vi "daq.vi"() -> ()   [LabVIEW 2010]
panel:
  in  "Array?":bool
  in  "Input":dbl format="%0.2f"
  in  "Tab Control":enum32{"DAQ"}(tab)
  out "Waveform DAQ":waveform(dbl)(graph)
  in  "Calibracion DAQ":T1
  in  "DAQ Controls":T2={"Minimum Value"=-10.0, "Maximum Value"=10.0, "Physical Channel"="Dev1/ao0", "DAQ Fs (S/s)"=10000.0} {"Minimum Value" min=-10.0 max=0.0; "Maximum Value" min=0.0 max=10.0}
  in  "tiempo (ms)":dbl
  in  "DAQ?":bool
  in  "stop":bool
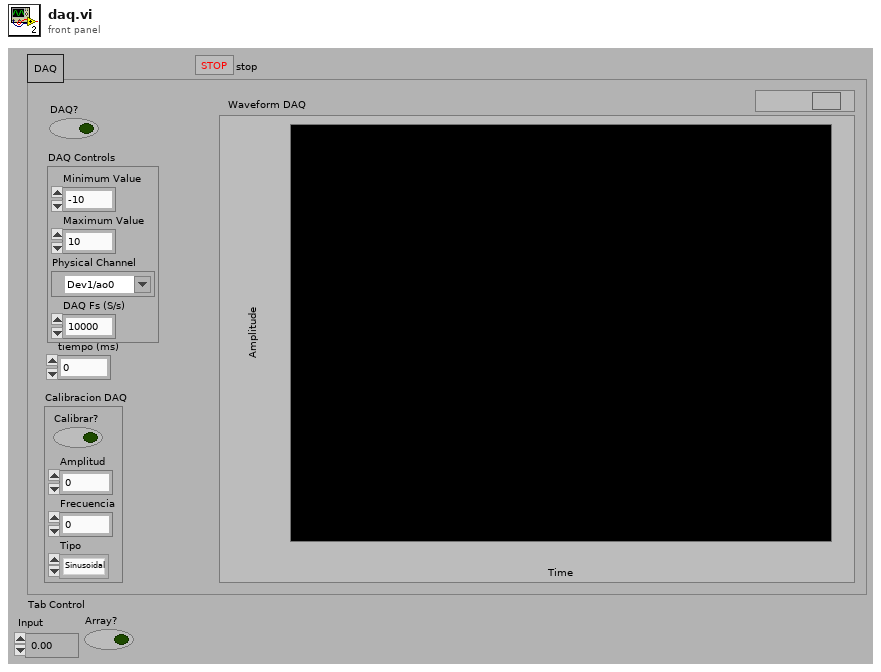
[diagram p1: front panel]
types:
  T1 = cluster{"Calibrar?":bool, "Amplitud":dbl, "Frecuencia":dbl, "Tipo":enum16{"Sinusoidal", "Triangular", "Cuadrada"}}
  T2 = cluster{"Minimum Value":dbl, "Maximum Value":dbl, "Physical Channel":tag, "DAQ Fs (S/s)":dbl}
  T3 = cluster{"DAQ Fs (S/s)":dbl, "task":refnum<k21>, "error":errorcluster, "Min Value":dbl, "Max Value":dbl}
  T4 = cluster{"DAQ Limits":cluster{"max":dbl, "min":dbl}, "Control Limits":cluster{"max":dbl, "min":dbl}}
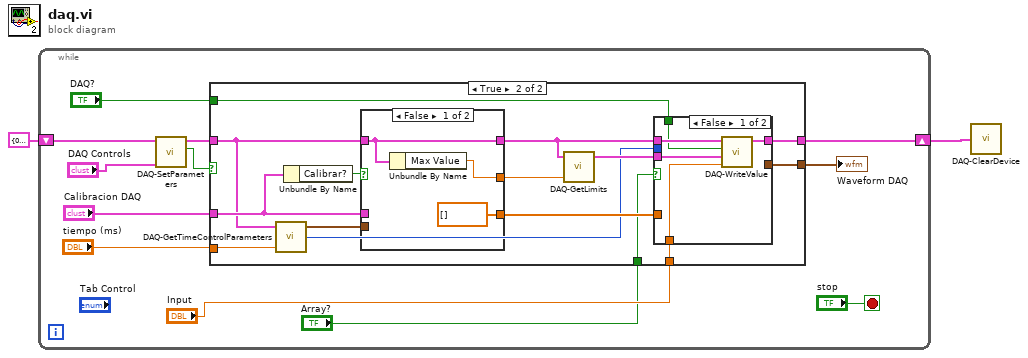
[diagram p0: block diagram]
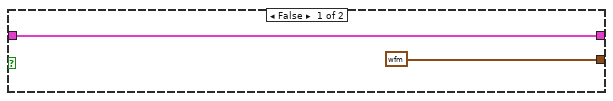
[diagram p2: hidden frame]
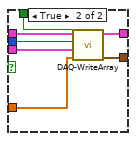
[diagram p3: hidden frame]
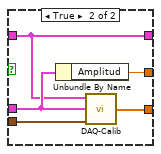
[diagram p4: hidden frame]
diagram:
  n1 = while {
    shift-right: [w6] -> w2
    shift-left: T3 {"DAQ Fs (S/s)"=0.0, "task"="", "error"={"status"=FALSE, "code"=0, "source"=""}, "Min Value"=0.0, "Max Value"=0.0} ("DAQ Device OUT") -> [w7]
    stop <- "stop" stop-if-true
    n2 = call "DAQ-SetParameters.vi"("DAQ Controls"="DAQ Controls", "DAQ Device IN"=w7) -> ("En Funcionamiento?"=w5:bool, "DAQ Device OUT"=w12:T3)  [unwired: 4 in]
    n3 = case shown="True" w5 {
      tunnel: "DAQ?" -> [_ w29]
      tunnel: w12 -> [w16 w20]
      tunnel: [waveform(dbl) {"t0"=timestamp(0 s since 1904-01-01), "dt"=1.0, "Y"=[]} ("Waveform Graph") w26] -> w11
      tunnel: "Calibracion DAQ" -> [_ w22]
      tunnel: "tiempo (ms)" -> [_ w24]
      tunnel: [w16 w23] -> w6
      tunnel: "Input" -> [_ w18]
      tunnel: "Array?" -> [_ w17]
      frame False {
      }
      frame True {
        n4 = call "DAQ-GetTimeControlParameters.vi"("tiempo (ms)"=w24, "DAQ Device IN"=w20) -> ("#samples"=w27:u32, "Time Control Parameters"=w28:cluster{"# samples":u32, "tiempos (ms)":dbl})  [unwired: 2 in]
        n5 = Unbundle By Name(w22) -> ("Calibrar?"=w21:bool)
        n6 = case shown="False" w21 {
          tunnel: [dbl[] [] ("Calibration OUT") w51] -> w31
          tunnel: w28 -> [_ w50]
          tunnel: w20 -> [w44 w47]
          tunnel: w22 -> [_ w49]
          tunnel: [w45 w48] -> w25
          tunnel: [w44 w47] -> w19
          frame False {
            n7 = Unbundle By Name(w44) -> ("Max Value"=w45:dbl)
          }
          frame True {
            n8 = Unbundle By Name(w49) -> ("Amplitud"=w48:dbl)
            n9 = call "DAQ-Calib.vi"("Time Control Parameters"=w50, "Calibracion DAQ"=w49, "DAQ Device IN"=w47) -> ("Calibration OUT"=w51:dbl[])  [unwired: 1 in]
          }
        }
        n10 = call "DAQ-GetLimits.vi"("Amplitud"=w25, "DAQ Device IN"=w19) -> ("Limites"=w30:T4)  [unwired: 3 in]
        n11 = case shown="False" w17 {
          tunnel: w31 -> [_ w43]
          tunnel: w30 -> [w33 w42]
          tunnel: w29 -> [w34 w41]
          tunnel: w27 -> [_ w40]
          tunnel: [_ w39] -> w26
          tunnel: [w35 w38] -> w23
          tunnel: w19 -> [w36 w37]
          tunnel: w18 -> [w32 _]
          frame False {
            n12 = call "DAQ-WriteValue.vi"("Input"=w32, "Limites"=w33, "DAQ?"=w34, "DAQ Device IN"=w36) -> ("DAQ Device OUT"=w35:T3)  [unwired: 5 in]
          }
          frame True {
            n13 = call "DAQ-WriteArray.vi"("DAQ?"=w41, "Control Array"=w43, "Limites"=w42, "#samples"=w40, "DAQ Device IN"=w37) -> ("Waveform Graph"=w39:waveform(dbl), "DAQ Device OUT"=w38:T3)  [unwired: 2 in]
          }
        }
      }
    }
    "Waveform DAQ" <- w11
  }
  n14 = call "DAQ-ClearDevice.vi"("DAQ Device IN"=w2) -> ()
